vi "Pfeiffer Vacuum OnTool Inert Gas System.vi"(8 "error in (no error)":errorcluster, 9 "PV OnTool Inert gas - Cluster":T1 {"Parameter" items=[" Sealing gas valve", " Flushing gas valve", " Gas ballast valve         ", " Direct control output K1   ", " Operating mode innert gas system", " Purge gas system OK  (read only)"]}, 10 "Adress of unit":u16=1 min=1 max=999 step=1, 11 "COM Port Name in":refnum<visa-resource-name>="COM1") -> (0 "error out":errorcluster, 1 "response (data)":string)   [LabVIEW 2016]
doc: "This VI is an example of how to use the Pfeiffer Vacuum subVIs programmatically. This VI first initializes the instrument, takes measurements, then closes the instrument."
uses:
  Public/OnTool/PV OnTool Inert Gas System - Cluster.ctl
  Pfeiffer Vacuum.lvlib
panel:
  # "Sealing gas valve                                       :\n Flushing gas valve                                     : \n Gas ballast valve                                        :\n Direct control output K1                           :\n Operating mode innert gas system        :"
  # "<--------------\n            off\n            off\n            off\n            off\n            automatic"
  # "----------->                \non  \non  \non  \non  \n              User control"
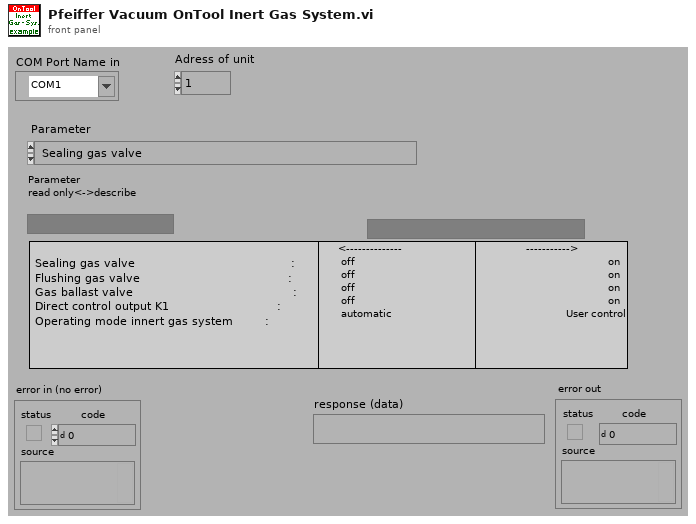
[diagram p1: front panel]
types:
  T1 = typedef "Pfeiffer Vacuum.lvlib/PV OnTool Inert Gas System - Cluster.ctl" = cluster{"Parameter":u16, "Parameter\nread only<->describe":bool, "off<->on":bool}
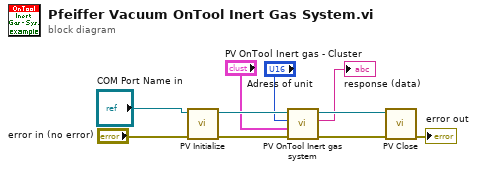
[diagram p0: block diagram]
diagram:
  n1 = call "PV Initialize.vi"("error in (no error)"="error in (no error)", "VISA session in"="COM Port Name in") -> ("error out"=w8:errorcluster, "VISA session out"=w6:refnum<visa-resource-name>)  [unwired: 8 in]
  n2 = call "PV OnTool Inert gas system.vi"("error in (no error)"=w8, "PV OnTool Inert gas - Cluster"="PV OnTool Inert gas - Cluster", "Adress of unit"="Adress of unit", "VISA session"=w6) -> ("error out"=w7:errorcluster, "response (data)"=→"response (data)":string, "dup VISA session"=w5:refnum<visa-resource-name>)  [unwired: 5 in]
  n3 = call "PV Close.vi"("VISA session"=w5, "error in (no error)"=w7) -> ("error out"=→"error out":errorcluster)  [unwired: 13 in]
